vi "Modify_Image_Thresholding_Settings-2.vi"(7 "[IN] Image Filtering Settings":T1, 8 "[IN] Index for thresholding":i8, 9 "[IN] Sigma":dbl min=0.1) -> (1 "[OUT] Image Filtering Settings":T1)   [LabVIEW 2017]
doc: "This subVI saves the sigma and thresholding index parameters into the cluster"
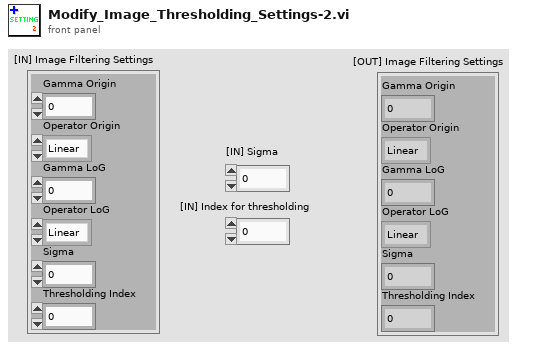
[diagram p1: front panel]
types:
  T1 = cluster{"Gamma Origin":sgl, "Operator Origin":enum32{"Linear", "Log", "Exp", "Square", "Square root", "Power X", "Power 1/X"}, "Gamma LoG":sgl, "Operator LoG":enum32{"Linear", "Log", "Exp", "Square", "Square root", "Power X", "Power 1/X"}, "Sigma":dbl, "Thresholding Index":i8}
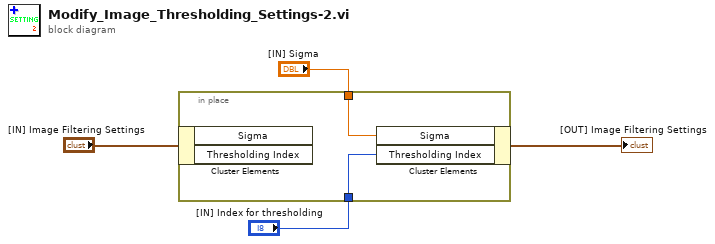
[diagram p0: block diagram]
diagram:
  n1 = in-place {
    in-place-border: "[IN] Sigma" -> [w6]
    in-place-border: "[IN] Index for thresholding" -> [w5]
    n2 = in-place-cluster #1("[IN] Image Filtering Settings") -> ()  [unwired: 2 out]
    n3 = in-place-cluster #1("Sigma"=w6, "Thresholding Index"=w5) -> (→"[OUT] Image Filtering Settings":T1)
  }
